vi "GetOpStateByName.vi"(10 "name":string, 11 "op state defs in":T1[](array[typedef])) -> (1 "found":bool, 2 "op state":T1, 3 "op state defs out":T1[](array[typedef]))   [LabVIEW 2017, in "DeviceModelHelpers.lvlib"]
uses:
  <vilib>/addons/InsightCM/Utilities/DeviceModelHelpers/DeviceModelHelpers.lvlib
  <vilib>/addons/InsightCM/MessageBus/Base/controls/ConfigListItem.ctl
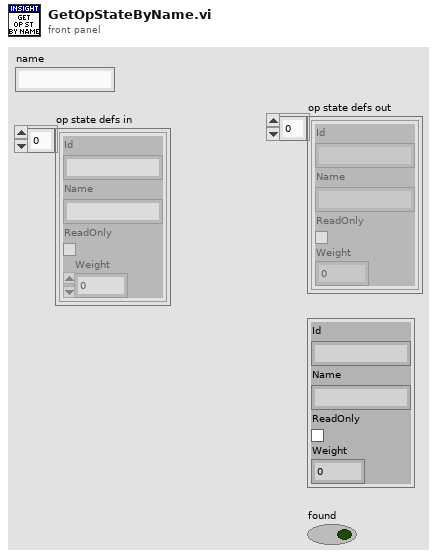
[diagram p1: front panel]
types:
  T1 = typedef "ConfigListItem.ctl" = cluster{"Id":string, "Name":string, "ReadOnly":bool, "Weight":i32}
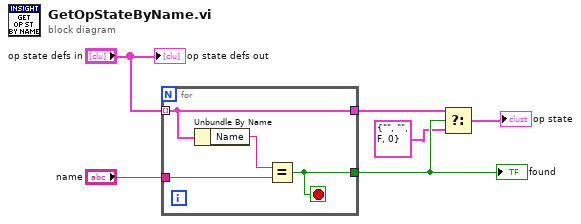
[diagram p0: block diagram]
diagram:
  n1 = for {
    tunnel: "op state defs in" -> [w8] mode=indexing
    tunnel: "name" -> [w9]
    tunnel: [w8] -> w5
    tunnel: [w7] -> w4
    stop <- w7 stop-if-true
    n2 = Unbundle By Name(w8) -> ("Name"=w10:string)
    n3 = Equal?(x=w10, y=w9) -> (x = y?=w7:bool)
  }
  "found" <- w4
  n4 = Select(t=w5, s=w4, f=T1 {"Id"="", "Name"="", "ReadOnly"=FALSE, "Weight"=0} ("op state 2")) -> (s? t:f=→"op state":T1)
  "op state defs out" <- "op state defs in"
